vi "Z.vi"(4 "Wire in":T1) -> (1 "Wire out":T1)   [LabVIEW 2016]
uses:
  TypeDefs/Circuit Cluster.ctl
  Classes/GateAbst/GateAbst.lvclass
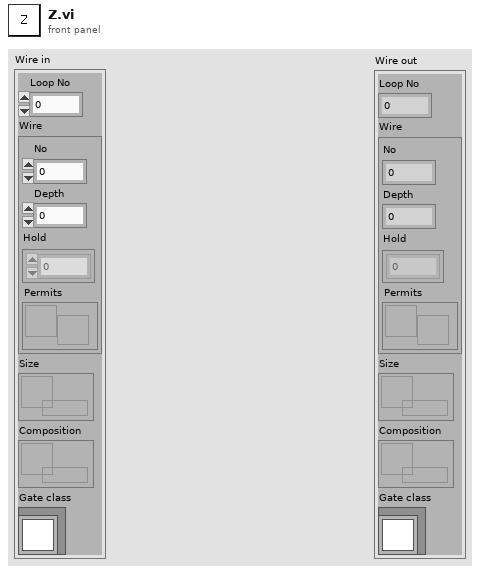
[diagram p1: front panel]
types:
  T1 = typedef "Circuit Cluster.ctl" = cluster{"Loop No":i32, "Wire":cluster{"No":i32, "Depth":i32, "Hold":i32[][], "Permits":refnum<notifier>}, "Size":refnum<queue>, "Composition":refnum<queue>, "Gate class":refnum<class "GateAbst.lvclass">}
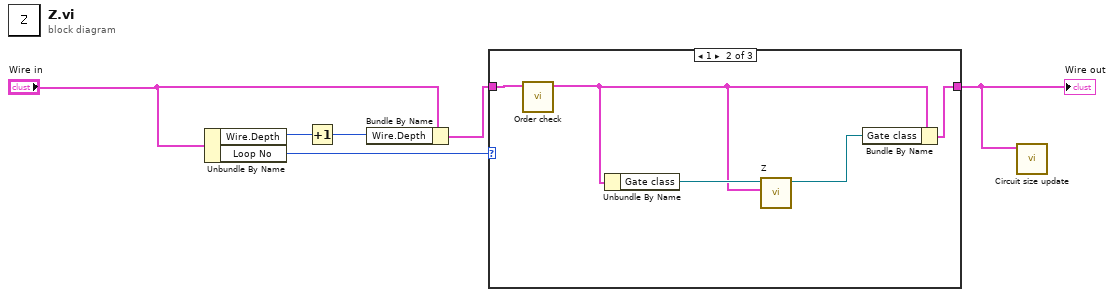
[diagram p0: block diagram]
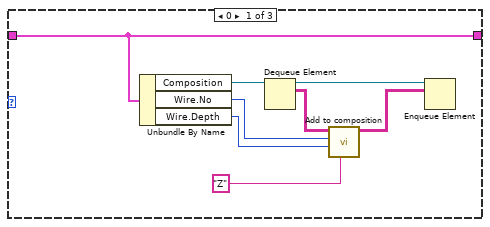
[diagram p2: hidden frame]
diagram:
  n1 = Unbundle By Name("Wire in") -> ("Wire.Depth"=w4:i32, "Loop No"=w1:i32)
  n2 = Increment(x=w4) -> (x+1=w5:i32)
  n3 = Bundle By Name(cluster="Wire in", "Wire.Depth"=w5) -> (w6:T1)
  n4 = case shown="1" w1 {
    tunnel: [w7 w18 w20] -> w2
    tunnel: w6 -> [w7 w15 w20]
    frame 0 {
      n5 = Unbundle By Name(w7) -> ("Composition"=w13:refnum<queue>, "Wire.No"=w9:i32, "Wire.Depth"=w8:i32)
      n6 = Dequeue Element(queue=w13) -> (queue out=w14:refnum<queue>, element=w10:string[][])  [unwired: 2 in, 2 out]
      n7 = call "Add to composition.vi"("Gate name"="Z", "Wire depth"=w8, "Wire No"=w9, "Composition in"=w10) -> ("Composition out"=w11:string[][])  [unwired: 7 in]
      n8 = Enqueue Element(queue=w14, element=w11) -> ()  [unwired: 2 in, 3 out]
    }
    frame 1 {
      n9 = call "Order check.vi"("Wire in in"=w15) -> ("Wire out"=w16:T1)  [unwired: 10 in]
      n10 = Unbundle By Name(w16) -> ("Gate class"=w19:refnum<class "GateAbst.lvclass">)
      n11 = call-dynamic "Z.vi"("Wire in"=w16, "GateAbst in"=w19) -> ("GateAbst out"=w17:refnum<class "GateAbst.lvclass">)  [unwired: 8 in, 1 out]
      n12 = Bundle By Name(cluster=w16, "Gate class"=w17) -> (w18:T1)
    }
    frame Default {
    }
  }
  "Wire out" <- w2
  n13 = call "Circuit size update.vi"("Wire in"=w2) -> ()  [unwired: 11 in]
